vi "grid spiral FGV.vi"(0 "X Step Size":fxp<+/-,24,16>, 1 "X Start":fxp<+/-,32,16>, 3 "Action":T2, 4 "Y Start":fxp<+/-,32,16>, 5 "Y Step Size":fxp<+/-,24,16>, 6 "X End":fxp<+/-,32,16>, 7 "Y End":fxp<+/-,32,16>, 8 "Det Frequency":fxp<+,32,0>=0.9999999997671694, 9 "Radial direction":T3=enum."Inward", 10 "Traj Frequency":fxp<+,32,0>=0.9999999997671694, 11 "Spiral Rotation Direction":T4) -> (12 "X-step":fxp<+/-,24,12>, 13 "Y-step":fxp<+/-,48,24>, 14 "X position":fxp<+/-,32,16>, 15 "Y position":fxp<+/-,32,16>, 16 "Direction arrays":T1[](array[typedef])=[enum."x up", enum."x up", enum."x up", enum."x up"], 17 "Steps array":i16[](array[numeric]), 18 "Number of positions":u32, 19 "Trajectory Complete":bool)   [LabVIEW 2015]
uses:
  spiral rotation direction.ctl
  spiral radial direction.ctl
  Trajectory FGV states.ctl
  grid spiral direction.ctl
  <vilib>/rvi/Emulation/niFpgaGetClockAttributes.vi
  <vilib>/rvi/Emulation/niFpgaSctlEmulationGetInTimedLoop.vi
  <vilib>/rvi/Emulation/niFpgaEmulationReportErrorSimple.vi
  <vilib>/rvi/Emulation/niFpgaCriticalErrorInLSC.vi
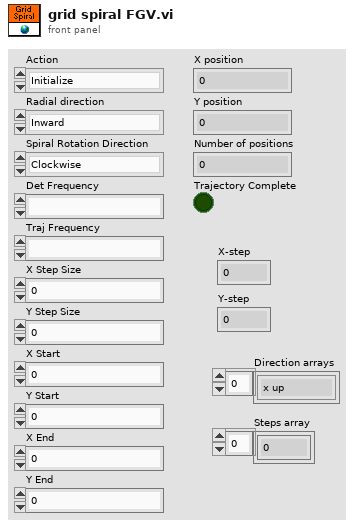
[diagram p1: front panel]
types:
  T1 = typedef "grid spiral direction.ctl" = enum16{"x up", "x down", "y up", "y down"}
  T2 = typedef "Trajectory FGV states.ctl" = enum16{"Initialize", "Increment"}
  T3 = typedef "spiral radial direction.ctl" = enum16{"Outward", "Inward"}
  T4 = typedef "spiral rotation direction.ctl" = enum16{"Clockwise", "Anti-clockwise"}
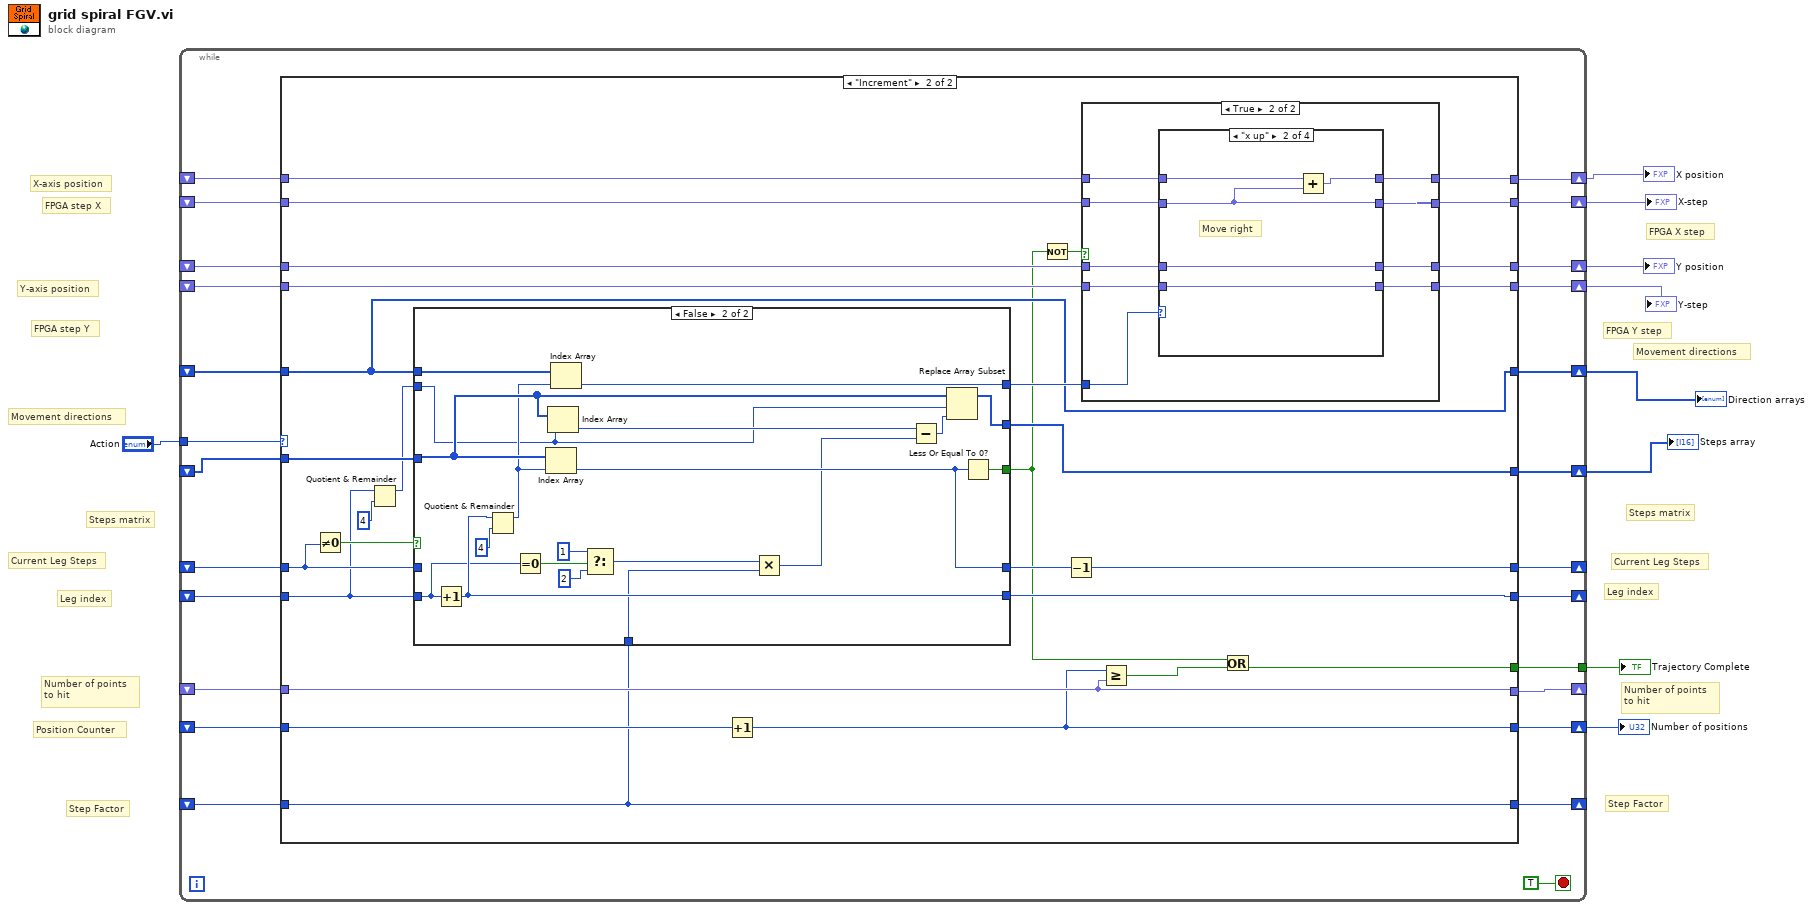
[diagram p0: block diagram]
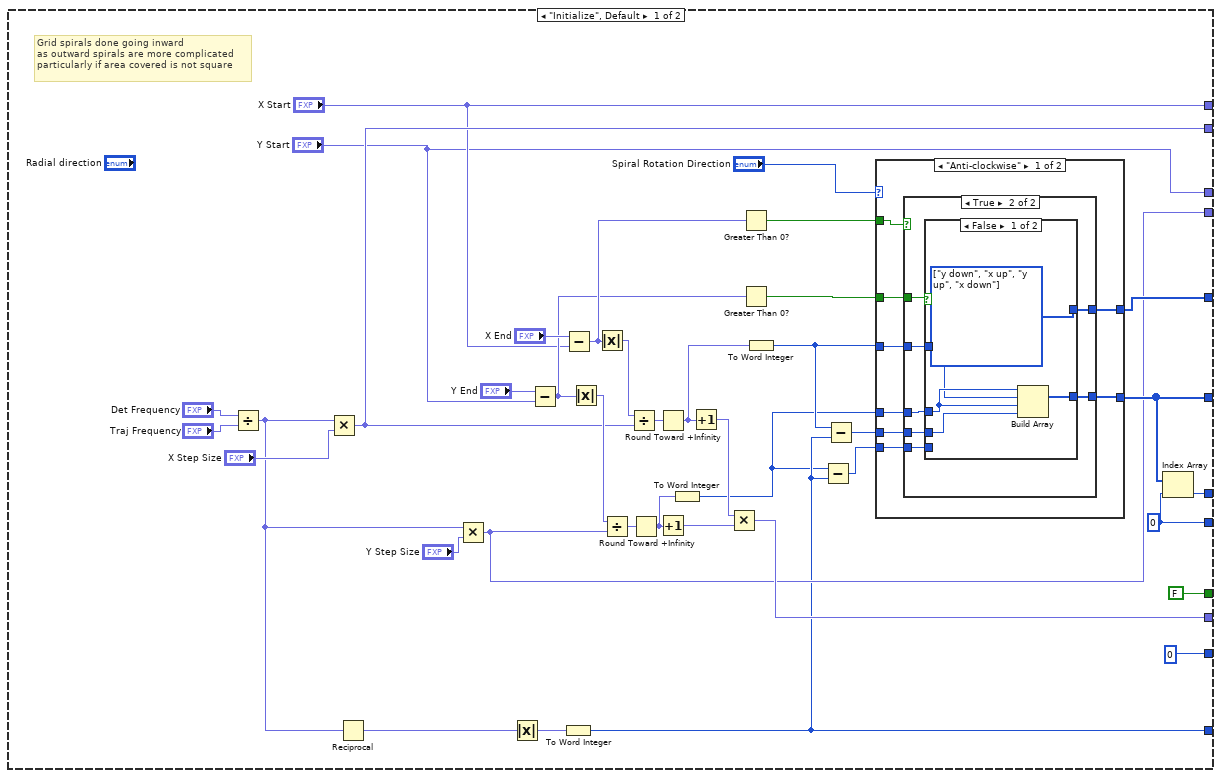
[diagram p2: hidden frame]
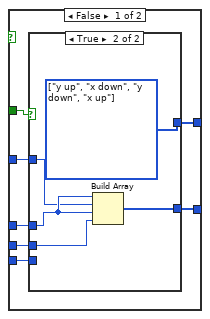
[diagram p3: hidden frame]
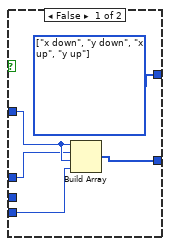
[diagram p4: hidden frame]
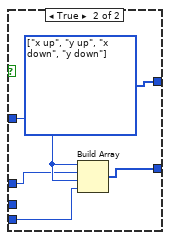
[diagram p5: hidden frame]
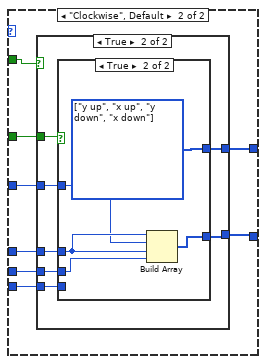
[diagram p6: hidden frame]
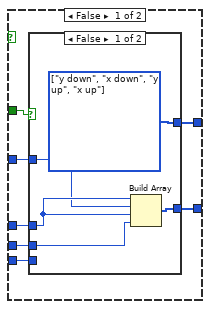
[diagram p7: hidden frame]
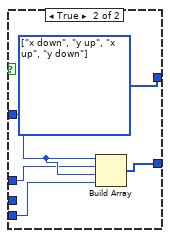
[diagram p8: hidden frame]
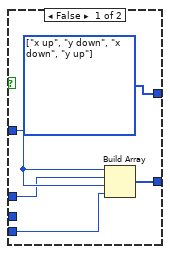
[diagram p9: hidden frame]
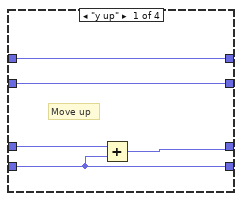
[diagram p11: hidden frame]
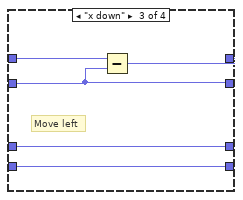
[diagram p12: hidden frame]
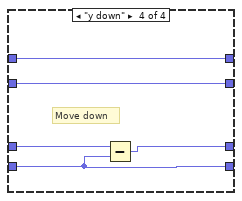
[diagram p13: hidden frame]
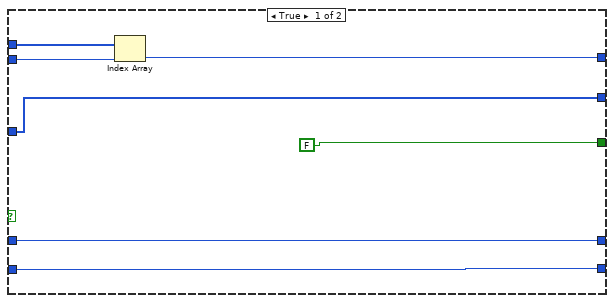
[diagram p14: hidden frame]
diagram:
  # "Step Factor"
  # "Step Factor"
  # "FPGA Y step"
  # "FPGA step Y"
  # "Current Leg Steps"
  # "Current Leg Steps"
  # "Leg index"
  # "Leg index"
  # "Steps matrix"
  # "Movement directions"
  # "Steps matrix"
  # "Movement directions"
  # "Number of points\nto hit"
  # "FPGA X step"
  # "Position Counter"
  # "X-axis position"
  # "Y-axis position"
  # "FPGA step X"
  # "Number of points\nto hit"
  n1 = while {
    tunnel: "Action" -> [w33]
    shift-right: [w16] -> w3
    shift-left: _ -> [w31]
    shift-right: [w30] -> _
    shift-left: _ -> [w29]
    shift-right: [w11] -> w6
    shift-left: _ -> [w28]
    shift-right: [w10] -> w5
    shift-left: _ -> [w32]
    tunnel: [w27] -> w8
    shift-right: [w26] -> w7
    shift-left: _ -> [w25]
    shift-right: [w23] -> w2
    shift-left: _ -> [w22]
    shift-right: [w24] -> w1
    shift-left: _ -> [w21]
    shift-right: [w19] -> _
    shift-left: _ -> [w20]
    shift-right: [w18] -> _
    shift-left: _ -> [w17]
    shift-right: [w15] -> w4
    shift-left: _ -> [w14]
    shift-right: [w13] -> _
    shift-left: _ -> [w12]
    stop <- TRUE stop-if-true
    n2 = case shown="\"Increment\"" w33 {
      tunnel: w28 -> [_ w176]
      tunnel: w32 -> [_ w174]
      tunnel: w31 -> [_ w173]
      tunnel: [w46 w171] -> w15
      tunnel: [w59 w168] -> w30
      tunnel: w29 -> [_ w168]
      tunnel: [FALSE w178] -> w27
      tunnel: [u32 0 w167] -> w26
      tunnel: w25 -> [_ w183]
      tunnel: [w49 w165] -> w24
      tunnel: [w52 w169] -> w23
      tunnel: w22 -> [_ w169]
      tunnel: w21 -> [_ w166]
      tunnel: w20 -> [_ w161]
      tunnel: [w50 w180] -> w19
      tunnel: [w48 w179] -> w18
      tunnel: w17 -> [_ w177]
      tunnel: [w45 w170] -> w16
      tunnel: w14 -> [_ w172]
      tunnel: [w41 w159] -> w13
      tunnel: w12 -> [_ w159]
      tunnel: ["X Start" w158] -> w11
      tunnel: ["Y Start" w157] -> w10
      frame "Initialize", Default {
        w50 = 0
        # "Grid spirals done going inward\nas outward spirals are more complicated\nparticularly if area covered is not square"
        n3 = Divide(x="Det Frequency", y="Traj Frequency") -> (x/y=w37:fxp<+,24,8>)
        n4 = Multiply(x=w37, y="X Step Size") -> (x*y=w45:fxp<+/-,24,12>)
        n5 = Reciprocal(x=w37) -> (1/x=w44:fxp<+,25,17>)
        n6 = Multiply(x=w37, y="Y Step Size") -> (x*y=w46:fxp<+/-,48,24>)
        n7 = Absolute Value(x=w44) -> (abs(x)=w43:fxp<+,25,17>)
        n8 = Subtract(x="Y End", y="Y Start") -> (x-y=w55:fxp<+/-,33,17>)
        n9 = To Word Integer(number=w43) -> (16bit integer=w41:i16)
        n10 = Subtract(x="X End", y="X Start") -> (x-y=w56:fxp<+/-,33,17>)
        n11 = Absolute Value(x=w55) -> (abs(x)=w65:fxp<+,32,16>)
        n12 = Absolute Value(x=w56) -> (abs(x)=w64:fxp<+,32,16>)
        n13 = Divide(x=w65, y=w46) -> (x/y=w63:fxp<+/-,64,41>)
        n14 = Divide(x=w64, y=w45) -> (x/y=w62:fxp<+/-,57,29>)
        n15 = Round Toward +Infinity(x=w63) -> (ceil(x): smallest int >= x=w57:fxp<+/-,42,42>)
        n16 = Round Toward +Infinity(x=w62) -> (ceil(x): smallest int >= x=w58:fxp<+/-,30,30>)
        n17 = Increment(x=w57) -> (x+1=w60:fxp<+/-,42,42>)
        n18 = To Word Integer(number=w57) -> (16bit integer=w40:i16)
        n19 = Increment(x=w58) -> (x+1=w61:fxp<+/-,30,30>)
        n20 = Multiply(x=w61, y=w60) -> (x*y=w59:fxp<+/-,64,70>)
        n21 = Greater Than 0?(x=w56) -> (x > 0?=w53:bool)
        n22 = Greater Than 0?(x=w55) -> (x > 0?=w54:bool)
        n23 = To Word Integer(number=w58) -> (16bit integer=w42:i16)
        n24 = Subtract(x=w40, y=w41) -> (x-y=w38:i16)
        n25 = Subtract(x=w42, y=w41) -> (x-y=w39:i16)
        n26 = case shown="\"Anti-clockwise\"" "Spiral Rotation Direction" {
          tunnel: w54 -> [w80 w122]
          tunnel: [w79 w121] -> w52
          tunnel: w42 -> [w77 w118]
          tunnel: w40 -> [w78 w119]
          tunnel: [w76 w120] -> w49
          tunnel: w53 -> [w75 w117]
          tunnel: w39 -> [w74 w116]
          tunnel: w38 -> [w73 w115]
          frame "Anti-clockwise" {
            n27 = case shown="True" w75 {
              tunnel: w80 -> [w87 w104]
              tunnel: [w86 w103] -> w79
              tunnel: w78 -> [w85 w101]
              tunnel: w77 -> [w84 w100]
              tunnel: [w83 w102] -> w76
              tunnel: w74 -> [w82 w99]
              tunnel: w73 -> [w81 w98]
              frame False {
                n28 = case shown="True" w87 {
                  tunnel: [w89 w94] -> w86
                  tunnel: w85 -> [w90 w97]
                  tunnel: w84 -> [w91 w95]
                  tunnel: [w92 w96] -> w83
                  tunnel: w82 -> [_ w93]
                  tunnel: w81 -> [w88 _]
                  frame False {
                    w89 = T1[] [enum."x down", enum."y down", enum."x up", enum."y up"] items=["x up", "x down", "y up", "y down"]
                    n29 = Build Array(w91, w90, w91, w88) -> (w92:i16[])
                  }
                  frame True {
                    w94 = T1[] [enum."y up", enum."x down", enum."y down", enum."x up"] items=["x up", "x down", "y up", "y down"]
                    n30 = Build Array(w97, w95, w97, w93) -> (w96:i16[])
                  }
                }
              }
              frame True {
                n31 = case shown="False" w104 {
                  tunnel: [w107 w112] -> w103
                  tunnel: [w109 w114] -> w102
                  tunnel: w101 -> [w108 w111]
                  tunnel: w100 -> [w106 w113]
                  tunnel: w99 -> [w105 _]
                  tunnel: w98 -> [_ w110]
                  frame False {
                    w107 = T1[] [enum."y down", enum."x up", enum."y up", enum."x down"] items=["x up", "x down", "y up", "y down"]
                    n32 = Build Array(w108, w106, w108, w105) -> (w109:i16[])
                  }
                  frame True {
                    w112 = T1[] [enum."x up", enum."y up", enum."x down", enum."y down"] items=["x up", "x down", "y up", "y down"]
                    n33 = Build Array(w113, w111, w113, w110) -> (w114:i16[])
                  }
                }
              }
            }
          }
          frame "Clockwise", Default {
            n34 = case shown="True" w117 {
              tunnel: w122 -> [w129 w146]
              tunnel: [w128 w145] -> w121
              tunnel: [w127 w144] -> w120
              tunnel: w119 -> [w126 w143]
              tunnel: w118 -> [w125 w142]
              tunnel: w116 -> [w124 w141]
              tunnel: w115 -> [w123 w140]
              frame False {
                n35 = case shown="False" w129 {
                  tunnel: [w132 w137] -> w128
                  tunnel: [w134 w139] -> w127
                  tunnel: w126 -> [w133 w136]
                  tunnel: w125 -> [w131 w138]
                  tunnel: w124 -> [w130 _]
                  tunnel: w123 -> [_ w135]
                  frame False {
                    w132 = T1[] [enum."y down", enum."x down", enum."y up", enum."x up"] items=["x up", "x down", "y up", "y down"]
                    n36 = Build Array(w133, w131, w133, w130) -> (w134:i16[])
                  }
                  frame True {
                    w137 = T1[] [enum."x down", enum."y up", enum."x up", enum."y down"] items=["x up", "x down", "y up", "y down"]
                    n37 = Build Array(w138, w136, w138, w135) -> (w139:i16[])
                  }
                }
              }
              frame True {
                n38 = case shown="True" w146 {
                  tunnel: [w149 w154] -> w145
                  tunnel: [w151 w156] -> w144
                  tunnel: w143 -> [w148 w155]
                  tunnel: w142 -> [w150 w153]
                  tunnel: w141 -> [_ w152]
                  tunnel: w140 -> [w147 _]
                  frame False {
                    w149 = T1[] [enum."x up", enum."y down", enum."x down", enum."y up"] items=["x up", "x down", "y up", "y down"]
                    n39 = Build Array(w150, w148, w150, w147) -> (w151:i16[])
                  }
                  frame True {
                    w154 = T1[] [enum."y up", enum."x up", enum."y down", enum."x down"] items=["x up", "x down", "y up", "y down"]
                    n40 = Build Array(w155, w153, w155, w152) -> (w156:i16[])
                  }
                }
              }
            }
          }
        }
        n41 = Index Array(array=w49, index=w50) -> (element=w48:i16)
      }
      frame "Increment" {
        n42 = Not Equal To 0?(x=w177) -> (x != 0?=w182:bool)
        n43 = Quotient & Remainder(x=w161, y=4) -> (x-y*floor(x/y)=w160:i32)  [unwired: 1 out]
        n44 = case shown="False" w182 {
          tunnel: w169 -> [w221 w240]
          tunnel: w166 -> [w220 w239]
          tunnel: w161 -> [w219 w230]
          tunnel: [w223 w243] -> w175
          tunnel: [w222 w242] -> w181
          tunnel: [w219 w235] -> w180
          tunnel: [FALSE w241] -> w164
          tunnel: w177 -> [w222 _]
          tunnel: [w220 w237] -> w165
          tunnel: w160 -> [w218 w225]
          tunnel: w159 -> [_ w227]
          frame True {
            n45 = Index Array(array=w221, index=w218) -> (element=w223:T1)
          }
          frame False {
            n46 = Increment(x=w230) -> (x+1=w235:i32)
            n47 = Quotient & Remainder(x=w235, y=4) -> (x-y*floor(x/y)=w234:i32)  [unwired: 1 out]
            n48 = Equal To 0?(x=w230) -> (x = 0?=w233:bool)
            n49 = Index Array(array=w239, index=w234) -> (element=w242:i16)
            n50 = Index Array(array=w239, index=w225) -> (element=w238:i16)
            n51 = Index Array(array=w240, index=w234) -> (element=w243:T1)
            n52 = Select(t=1, s=w233, f=2 ("y")) -> (s? t:f=w228:i32)
            n53 = Multiply(x=w228, y=w227) -> (x*y=w229:i32)
            n54 = Subtract(x=w238, y=w229) -> (x-y=w226:i32)
            n55 = Replace Array Subset(array=w239, new element=w226, index=w225) -> (w237:i16[])
            n56 = Less Or Equal To 0?(x=w242) -> (x <= 0?=w241:bool)
          }
        }
        n57 = Increment(x=w183) -> (x+1=w167:u32)
        n58 = Not(x=w164) -> (.not. x?=w163:bool)
        n59 = Decrement(x=w181) -> (x-1=w179:i16)
        n60 = case shown="True" w163 {
          tunnel: w176 -> [w188 w197]
          tunnel: w175 -> [_ w196]
          tunnel: w174 -> [w186 w195]
          tunnel: w173 -> [w187 w194]
          tunnel: w172 -> [w185 w193]
          tunnel: [w185 w192] -> w171
          tunnel: [w186 w191] -> w157
          tunnel: [w187 w190] -> w170
          tunnel: [w188 w189] -> w158
          frame False {
          }
          frame True {
            n61 = case shown="\"x up\"" w196 {
              tunnel: w197 -> [w201 w207 w212 w216]
              tunnel: w194 -> [w200 w205 w209 w215]
              tunnel: w195 -> [w202 w206 w211 w217]
              tunnel: w193 -> [w199 w204 w210 w214]
              tunnel: [w198 w206 w211 w213] -> w191
              tunnel: [w201 w203 w208 w216] -> w189
              tunnel: [w200 w205 w209 w215] -> w190
              tunnel: [w199 w204 w210 w214] -> w192
              frame "y up" {
                # "Move up"
                n62 = Add(x=w202, y=w199) -> (x+y=w198:fxp<+/-,32,16>)
              }
              frame "x up" {
                # "Move right"
                n63 = Add(x=w207, y=w205) -> (x+y=w203:fxp<+/-,32,16>)
              }
              frame "x down" {
                # "Move left"
                n64 = Subtract(x=w212, y=w209) -> (x-y=w208:fxp<+/-,32,16>)
              }
              frame "y down" {
                # "Move down"
                n65 = Subtract(x=w217, y=w214) -> (x-y=w213:fxp<+/-,32,16>)
              }
            }
          }
        }
        n66 = Greater Or Equal?(x=w167, y=w168) -> (x >= y?=w184:bool)
        n67 = Or(x=w164, y=w184) -> (x .or. y?=w178:bool)
      }
    }
  }
  "Number of positions" <- w7
  "X position" <- w6
  "Y position" <- w5
  "Trajectory Complete" <- w8
  "Y-step" <- w4
  "X-step" <- w3
  "Steps array" <- w1
  "Direction arrays" <- w2
